vi "Ctrl.ListBox.StyleFont.vi"(8 "error in (no error)":errorcluster, 10 "Font Info":T1, 11 "Listbox Ref":refnum<vi>) -> (0 "error out":errorcluster, 3 "Listbox Ref out":refnum<vi>)   [LabVIEW 2020]
uses:
  Font Info -- Cluster.ctl
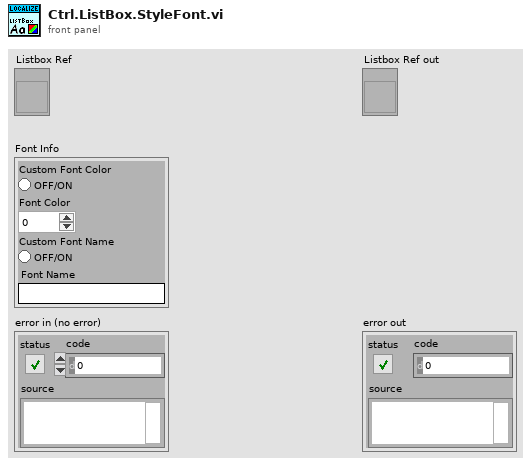
[diagram p1: front panel]
types:
  T1 = typedef "Font Info -- Cluster.ctl" = cluster{"Custom Font Color":bool, "Font Color":u32, "Custom Font Name":bool, "Font Name":string}
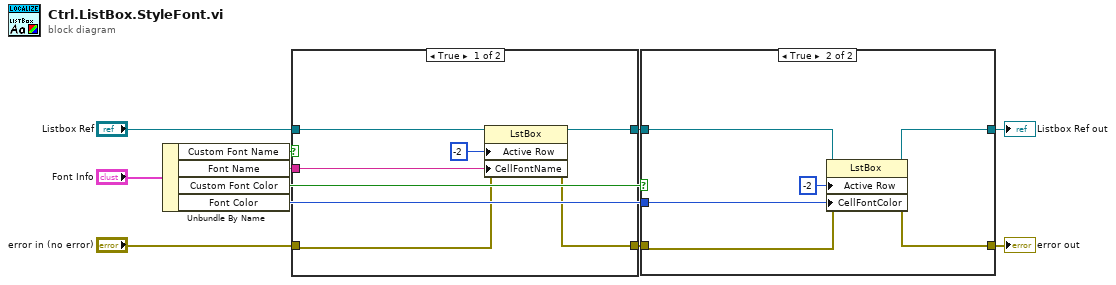
[diagram p0: block diagram]
diagram:
  n1 = Unbundle By Name("Font Info") -> ("Custom Font Name"=w10:bool, "Font Name"=w5:string, "Custom Font Color"=w8:bool, "Font Color"=w4:u32)
  n2 = case shown="True" w10 {
    tunnel: [w12 w19] -> w9
    tunnel: "error in (no error)" -> [w13 w19]
    tunnel: w5 -> [w16 _]
    tunnel: "Listbox Ref" -> [w15 w18]
    tunnel: [w14 w18] -> w2
    frame True {
      n3 = property class="LstBox"(reference=w15, error in=w13, "Active Row"=-2 ("Active Row:Active Row Number"), "CellFontName"=w16) -> (reference out=w14:refnum<vi>, error out=w12:errorcluster)
    }
    frame False {
    }
  }
  n4 = case shown="True" w8 {
    tunnel: w9 -> [w21 w23]
    tunnel: [w21 w22] -> w6
    tunnel: w4 -> [_ w25]
    tunnel: w2 -> [w20 w27]
    tunnel: [w20 w26] -> w1
    frame False {
    }
    frame True {
      n5 = property class="LstBox"(reference=w27, error in=w23, "Active Row"=-2 ("Active Row:Active Row Number"), "CellFontColor"=w25) -> (reference out=w26:refnum<vi>, error out=w22:errorcluster)
    }
  }
  "error out" <- w6
  "Listbox Ref out" <- w1
